vi "Read Justification.vi"(9 "Text in":refnum<class "Text.lvclass">) -> (3 "Text out":refnum<class "Text.lvclass">, 4 "Justification":enum16{"Left", "Center", "Right"}(ring))   [LabVIEW 2014, in "Text.lvclass"]
uses:
  Text.lvclass
  Text.lvclass/Text.ctl
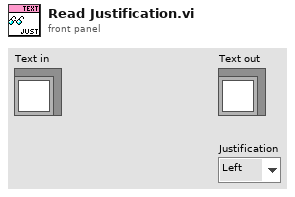
[diagram p1: front panel]
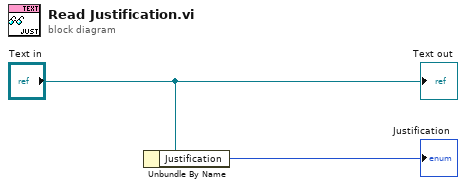
[diagram p0: block diagram]
diagram:
  n1 = Unbundle By Name("Text in") -> ("Justification"=→"Justification":enum16{"Left", "Center", "Right"})
  "Text out" <- "Text in"
